vi "题目1.vi"() -> ()   [LabVIEW 2017]
panel:
  out "波形图表 2":dbl[](graph)
  in  "滑动杆 2":dbl(slide) scale=0.0..10.0
  out "波形图表":dbl(graph)
  in  "滑动杆":dbl(slide) scale=0.0..10.0
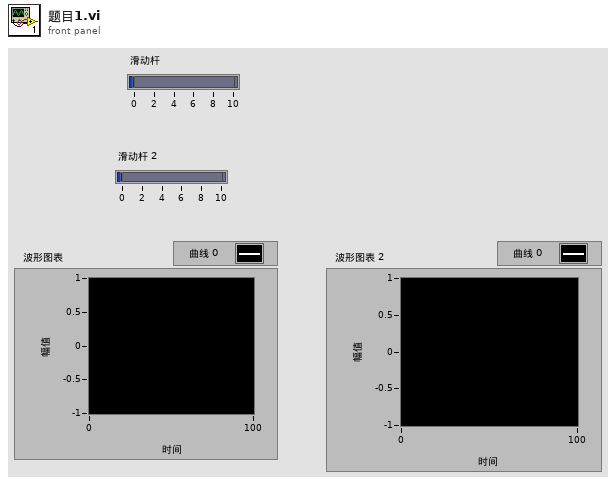
[diagram p1: front panel]
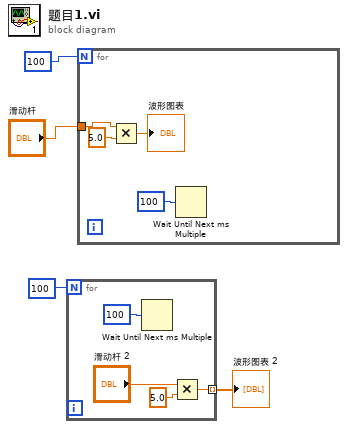
[diagram p0: block diagram]
diagram:
  n1 = for {
    N: 100 -> [_]
    tunnel: [w6] -> w1 mode=indexing
    n2 = Wait Until Next ms Multiple(millisecond multiple=100) -> ()  [unwired: 1 out]
    n3 = Multiply(x="滑动杆 2", y=5.0) -> (x*y=w6:dbl)
  }
  "波形图表 2" <- w1
  n4 = for {
    N: 100 -> [_]
    tunnel: "滑动杆" -> [w11]
    n5 = Multiply(x=w11, y=5.0) -> (x*y=→"波形图表":dbl)
    n6 = Wait Until Next ms Multiple(millisecond multiple=100) -> ()  [unwired: 1 out]
  }
